vi "Hall DC.vi"() -> ()   [LabVIEW 2018]
panel:
  in  "Y chan":i32=3
  out "XY Graph 3":T1(graph)
  in  "X coumn index":i32
  in  "File 2":path
  in  "Flatness":dbl=0.05
  out "R Hall mean":dbl
  out "XY Graph 2":cluster{"Field":dbl[], dbl[]}[](graph)
  in  "Bin size":dbl=0.1
  out "XY Graph":cluster{dbl[], dbl[]}[](graph)
  in  "Signal channel":string="LakeShore 370 (20) R"
  in  "Field channel":string="IPS120 (25) Field"
  in  "Group":string="p"
  in  "File 1":path
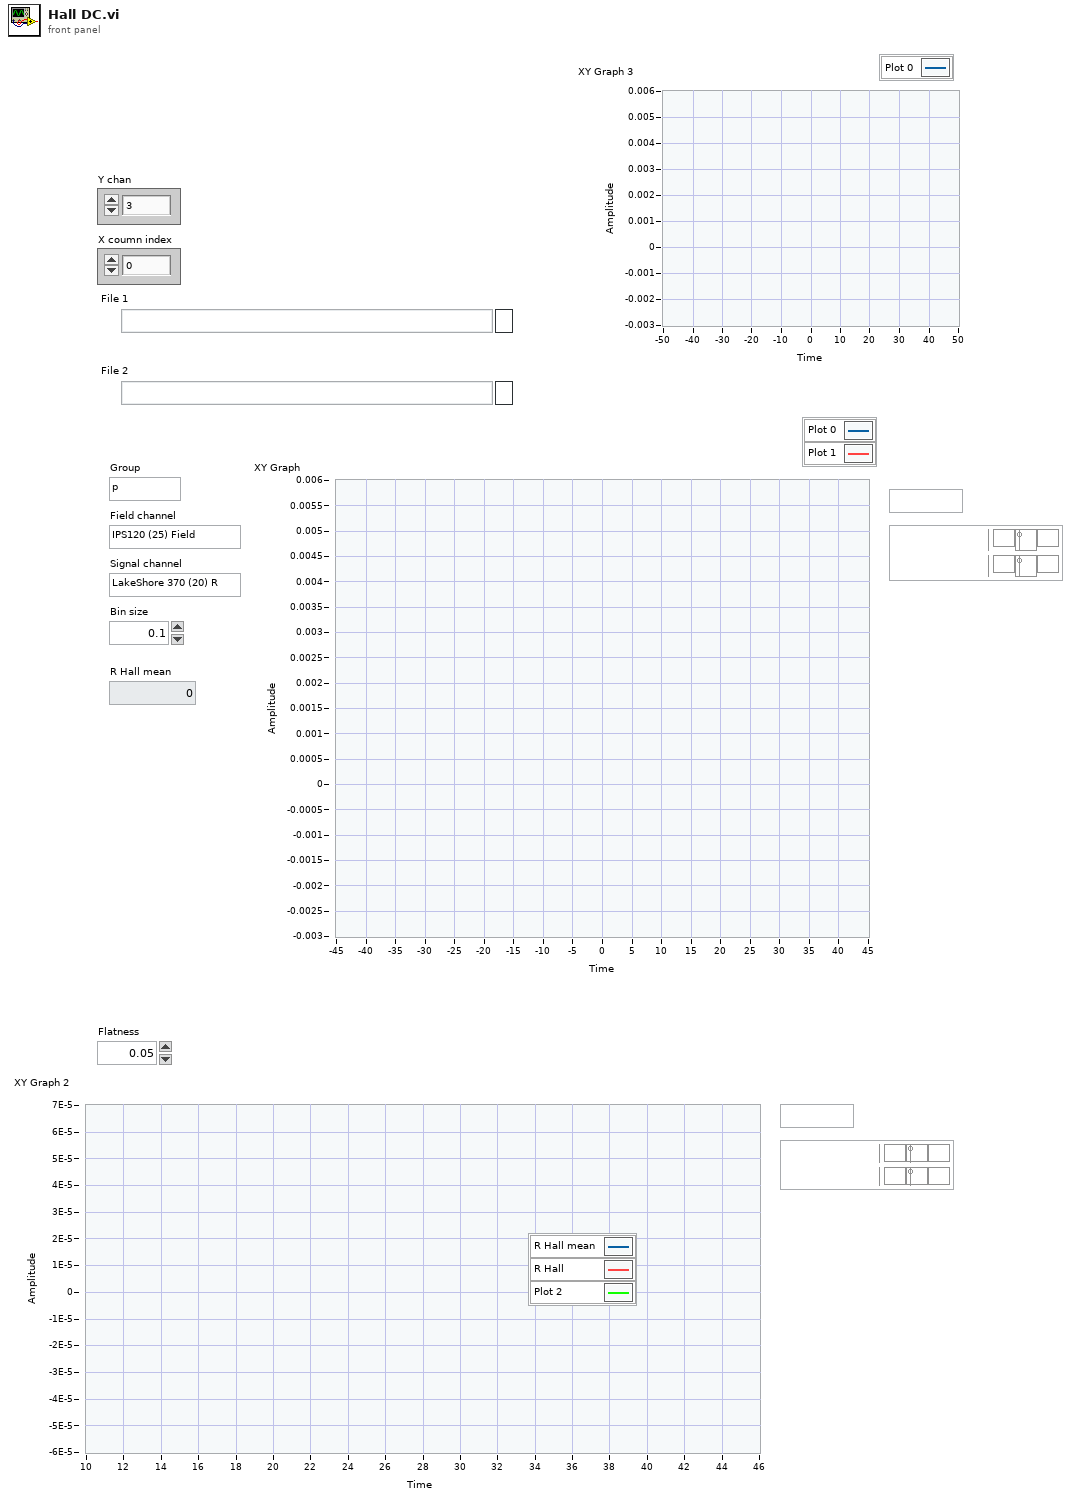
[diagram p1: front panel]
types:
  T1 = cluster{"Binned data":dbl[], "Binned data":dbl[]}
  T2 = enum16{"open", "open or create", "create or replace", "create", "open (read-only)"}
  T3 = cluster{"Binned data":dbl[], "Binned data":dbl[]}[]
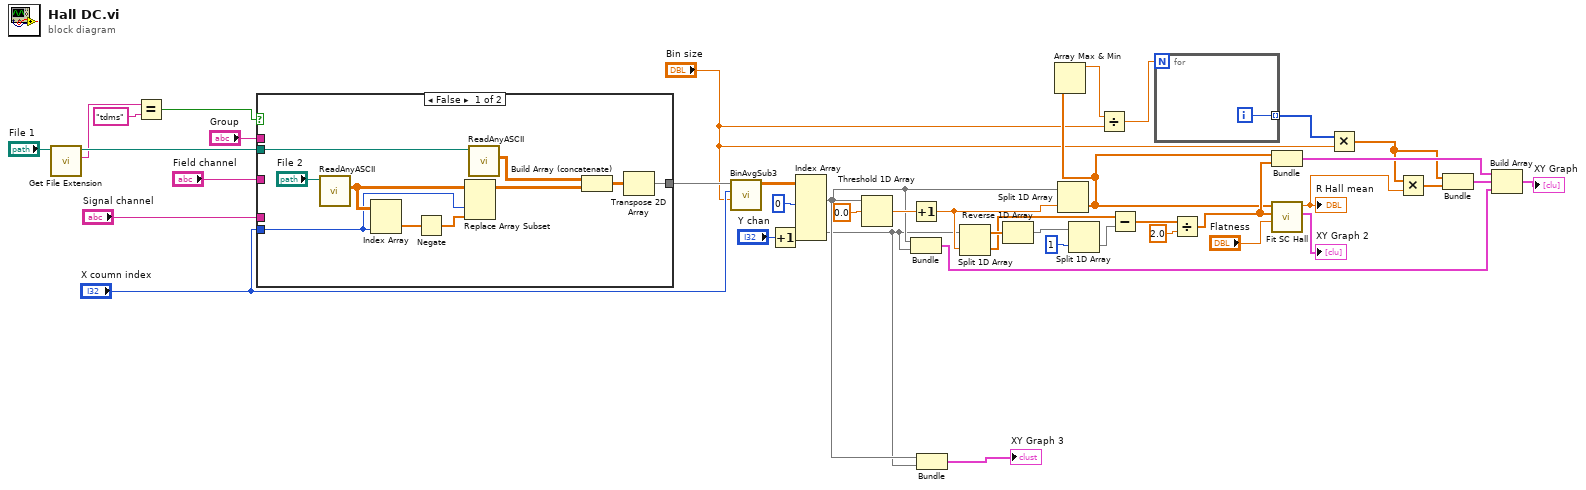
[diagram p0: block diagram]
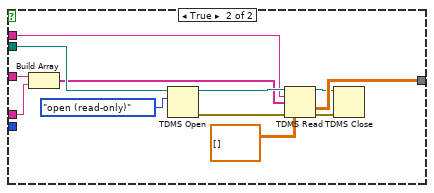
[diagram p2: hidden frame]
diagram:
  n1 = call <vilib>:"Get File Extension.vi"("file"="File 1") -> ("lowercase file extension"=w15:string, "dup file"=w16:path)  [unwired: 6 in, 3 out]
  n2 = Equal?(x=w15, y="tdms") -> (x = y?=w13:bool)
  n3 = case shown="False" w13 {
    tunnel: w16 -> [w52 w64]
    tunnel: "Group" -> [_ w60]
    tunnel: "Field channel" -> [_ w59]
    tunnel: "Signal channel" -> [_ w57]
    tunnel: [w44 w55] -> w39
    tunnel: "X coumn index" -> [w48 _]
    frame False {
      n4 = call "ReadAnyASCII.vi"("file path (dialog if empty)"="File 2") -> ("all rows"=w49:dbl[][])  [unwired: 8 in, 2 out]
      n5 = Index Array(array=w49, index (col)=w48) -> (element=w50:dbl[])  [unwired: 1 in]
      n6 = Negate(x=w50) -> (-x=w43:dbl[])
      n7 = Replace Array Subset(array=w49, new element=w43, index (col)=w48) -> (w46:dbl[][])  [unwired: 1 in]
      n8 = call "ReadAnyASCII.vi"("file path (dialog if empty)"=w52) -> ("all rows"=w47:dbl[][])  [unwired: 8 in, 2 out]
      n9 = Build Array (concatenate)(w47, w46) -> (w45:dbl[][])
      n10 = Transpose 2D Array(2D array=w45) -> (transposed array=w44:dbl[][])
    }
    frame True {
      n11 = Build Array(w59, w57) -> (w58:string[])
      n12 = TDMS Open(10:T2."open (read-only)" ("operation (0:open)"), 11:w64) -> (0:w61:errorcluster, 3:w62:refnum<k34>)  [unwired: 5 in]
      n13 = TDMS Read(0:w62, 5:w60, 7:w58, 11:w61, 12:dbl[][] []) -> (4:w53:refnum<k34>, 10:w55:dbl[][], 15:w54:errorcluster)  [unwired: 3 in, 3 out]
      n14 = TDMS Close(8:w54, 11:w53) -> ()  [unwired: 2 out]
    }
  }
  n15 = call "BinAvgSub3.vi"("Bin size"="Bin size", "X coumn index"="X coumn index", "Data in"=w39) -> ("Binned data"=w37:dbl[][])  [unwired: 2 in, 6 out]
  n16 = Increment(x="Y chan") -> (x+1=w6:i32)
  n17 = Index Array(array=w37, index (col) #1=0 ("disabled index (col)"), index (col) #3=w6) -> (element #1=w10:dbl[], element #3=w8:dbl[])  [unwired: 4 in, 1 out]
  n18 = Threshold 1D Array(2:0.0 ("element"), 3:w10) -> (0:w33:dbl)  [unwired: 1 in]
  n19 = Increment(x=w33) -> (x+1=w32:dbl)
  n20 = Bundle("Binned data"=w10, "Binned data"=w8) -> (w36:T1)  [unwired: 1 in]
  n21 = Bundle("Binned data"=w10, "Binned data"=w8) -> (→"XY Graph 3":T1)  [unwired: 1 in]
  n22 = Split 1D Array(array=w8, index=w32) -> (first subarray=w31:dbl[], second subarray=w28:dbl[])
  n23 = Reverse 1D Array(array=w31) -> (reversed array=w30:dbl[])
  n24 = Split 1D Array(array=w10, index=w32) -> (second subarray=w5:dbl[])  [unwired: 1 out]
  n25 = Array Max & Min(array=w5) -> (max value=w4:dbl)  [unwired: 3 out]
  n26 = Split 1D Array(array=w30, index=1) -> (second subarray=w27:dbl[])  [unwired: 1 out]
  n27 = Divide(x=w4, y="Bin size") -> (x/y=w2:dbl)
  n28 = Subtract(x=w28, y=w27) -> (x-y=w21:dbl[])
  n29 = for {
    N: w2 -> [_]
    tunnel: [w65] -> w26 mode=indexing
    i -> [w65]
  }
  n30 = Divide(x=w21, y=2.0) -> (x/y=w22:dbl[])
  n31 = Bundle(w5, w22) -> (w25:cluster{dbl[], dbl[]})  [unwired: 1 in]
  n32 = call "Fit SC Hall.vi"("Flatness"="Flatness", "Hall signal"=w22, "Field"=w5) -> ("XY Graph"=→"XY Graph 2":cluster{"Field":dbl[], dbl[]}[], "Mean"=w18:dbl)  [unwired: 7 in]
  "R Hall mean" <- w18
  n33 = Multiply(x=w26, y="Bin size") -> (x*y=w1:dbl[])
  n34 = Multiply(x=w1, y=w18) -> (x*y=w23:dbl[])
  n35 = Bundle(w1, w23) -> (w24:cluster{dbl[], dbl[]})  [unwired: 1 in]
  n36 = Build Array(w25, w24, w36) -> (→"XY Graph":T3)
